vi "InitializeLithographyObject.vi"(8 "error in (no error)":errorcluster, 11 "Asylum_Driver in":refnum<class "Asylum_Driver.lvclass">) -> (0 "error out":errorcluster, 3 "Asylum_Driver out":refnum<class "Asylum_Driver.lvclass">)   [LabVIEW 2019, in "Asylum_Driver.lvclass"]
uses:
  Asylum_Driver.lvclass
  AFM Driver/AFM_Driver.lvclass
  C:/Users/Albro/Documents/GitHub/AFM-Lithography/lvsrc/AFMs/AFM Driver/AFM_Driver.lvclass
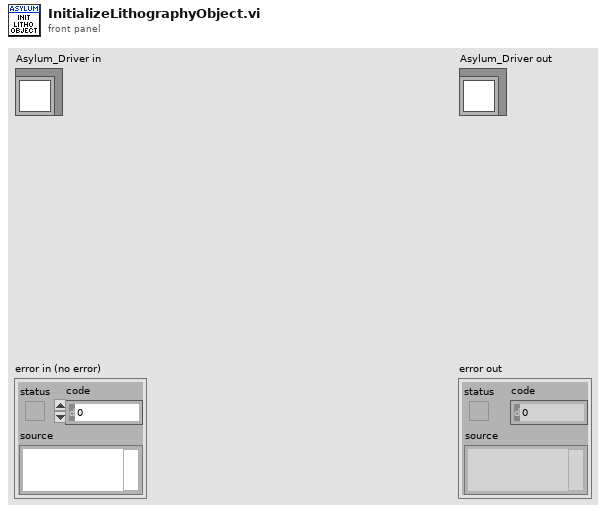
[diagram p1: front panel]
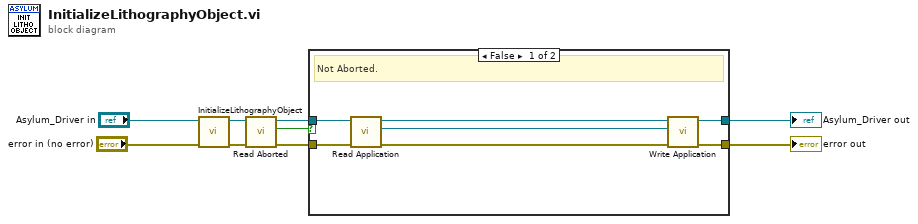
[diagram p0: block diagram]
diagram:
  n1 = call-parent "InitializeLithographyObject.vi"("error in (no error)"="error in (no error)", "AFM_Driver in"="Asylum_Driver in") -> ("error out"=w1:errorcluster, "AFM_Driver out"=w4:refnum<class "Asylum_Driver.lvclass">)  [unwired: 8 in]
  n2 = call "Read Aborted.vi"("error in (no error)"=w1, "AFM_Driver in"=w4) -> ("error out"=w5:errorcluster, "Aborted?"=w7:bool, "AFM_Driver out"=w6:refnum<class "Asylum_Driver.lvclass">)  [unwired: 7 in]
  n3 = case shown="False" w7 {
    tunnel: w6 -> [w14 w18]
    tunnel: [w15 w18] -> w3
    tunnel: [w12 w17] -> w2
    tunnel: w5 -> [w11 w17]
    frame False {
      # "Not Aborted."
      n4 = call-dynamic "Read Application.vi"("error in (no error)"=w11, "Asylum_Driver in"=w14) -> ("error out"=w13:errorcluster, "Application"=w10:refnum<k7>, "Asylum_Driver out"=w16:refnum<class "Asylum_Driver.lvclass">)  [unwired: 7 in]
      n5 = call-dynamic "Write Application.vi"("error in (no error)"=w13, "Application"=w10, "Asylum_Driver in"=w16) -> ("error out"=w12:errorcluster, "Asylum_Driver out"=w15:refnum<class "Asylum_Driver.lvclass">)  [unwired: 7 in]
    }
    frame True {
      # "Aborted. This state must stay empty."
    }
  }
  "error out" <- w2
  "Asylum_Driver out" <- w3
